vi "Get configuration chain.vi"(8 "error in (no error)":errorcluster, 11 "ConfocalStageBase in":refnum<class "ConfocalStage.lvclass">) -> (0 "error out":errorcluster, 1 "class name":string[](array[string]), 2 "configuration chain":variant[](array[variant]), 3 "ConfocalStageBase out":refnum<class "ConfocalStage.lvclass">)   [LabVIEW 2012, in "ConfocalStage.lvclass"]
doc: "Returns an array of variants containing the configuration clusters of each class in the inheritance chain (lowest child class first), together with an array of all class names in the inheritance chain.\n\nFor classes without configuration cluster, the configuration chain contains empty variants."
uses:
  ConfocalStage.lvclass
  <vilib>/Distrio/Murmex/Murmex/Murmex.lvclass
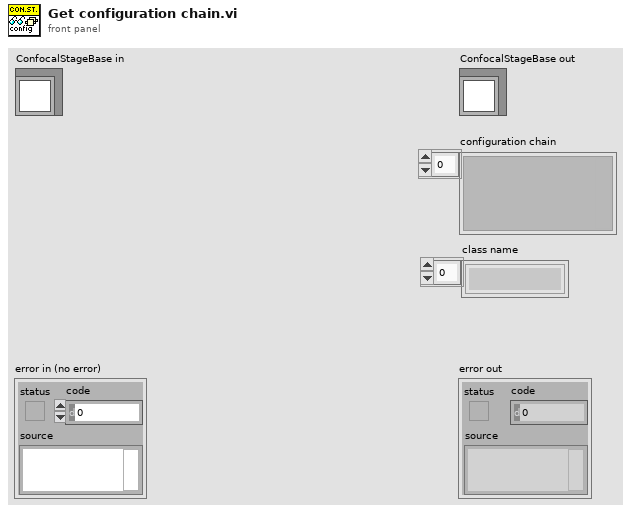
[diagram p1: front panel]
types:
  T1 = typedef "ConfocalStage.lvclass/configuration.ctl" = cluster{"startup speed":dbl[unit], "Serial port":cluster{"baud rate":u32, "data bits":u16, "parity (0:none)":enum16{"None", "Odd", "Even", "Mark", "Space"}, "flow control":u16, "stop bits":u16, "termination char":u8, "send termination char?":bool, "COM port":refnum<visa-resource-name>}, "accelleration ramp":dbl[unit], "speed conversion":dbl, "position conversion X":dbl, "position conversion Y":dbl, "position conversion Z":dbl}
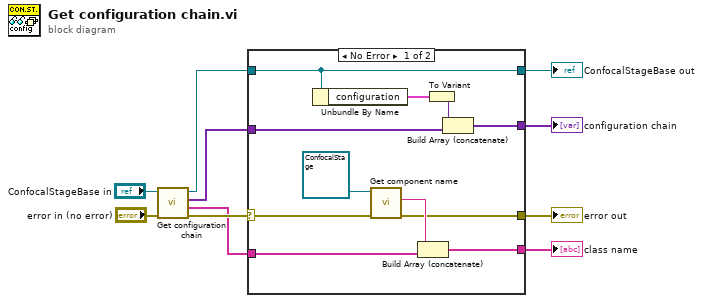
[diagram p0: block diagram]
diagram:
  n1 = call-parent "Get configuration chain.vi"("error in (no error)"="error in (no error)", "MurmexBase in"="ConfocalStageBase in") -> ("error out"=w8:errorcluster, "class name"=w2:string[], "configuration chain"=w4:variant[], "MurmexBase out"=w5:refnum<class "ConfocalStage.lvclass">)  [unwired: 6 in]
  n2 = case shown="No Error" w8 {
    selector: w8 -> [w18 w22]
    tunnel: [w17 w22] -> w7
    tunnel: [w16 w23] -> w6
    tunnel: w5 -> [w16 w23]
    tunnel: w4 -> [w15 _]
    tunnel: [w14 _] -> w3
    tunnel: w2 -> [w13 _]
    tunnel: [w12 _] -> w1
    frame No Error {
      n3 = Unbundle By Name(w16) -> ("configuration"=w21:T1)
      n4 = call <vilib>:"Get component name.vi"("error in (no error)"=w18, "Murmex in"=refnum<class "ConfocalStage.lvclass"> refnum ("ConfocalStageBase in")) -> ("error out"=w17:errorcluster, "component name"=w19:string)  [unwired: 7 in, 1 out]
      n5 = Build Array (concatenate)(w19, w13) -> (w12:string[])
      n6 = To Variant(anything=w21) -> (Variant=w20:variant)
      n7 = Build Array (concatenate)(w20, w15) -> (w14:variant[])
    }
    frame Error {
    }
  }
  "error out" <- w7
  "ConfocalStageBase out" <- w6
  "configuration chain" <- w3
  "class name" <- w1
